vi "Close.vi"(8 "error in (no error)":errorcluster, 11 "IKA EUROSTAR Settings":T1) -> (0 "error out":errorcluster, 3 "IKA EUROSTAR Settings":T1)   [LabVIEW 2018, in "IKA EUROSTAR.lvlib"]
uses:
  IKA EUROSTAR.lvlib
  IKA EUROSTAR Settings.ctl
  support/Support Library.lvlib
panel:
  out "read buffer 2":string
  out "read buffer":string
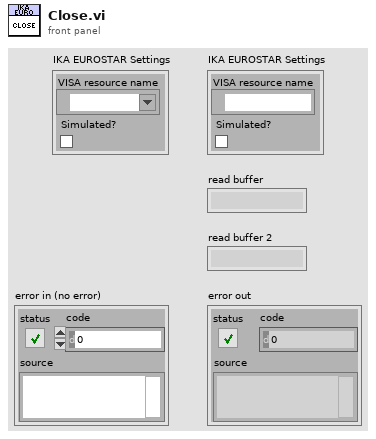
[diagram p1: front panel]
types:
  T1 = typedef "IKA EUROSTAR.lvlib/IKA EUROSTAR Settings.ctl" = cluster{"VISA resource name":refnum<visa-resource-name>, "Simulated?":bool}
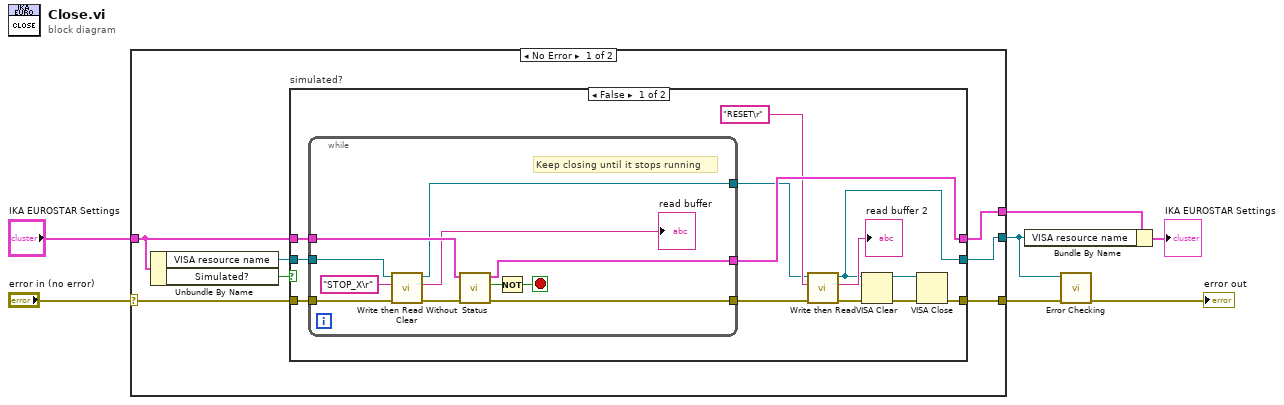
[diagram p0: block diagram]
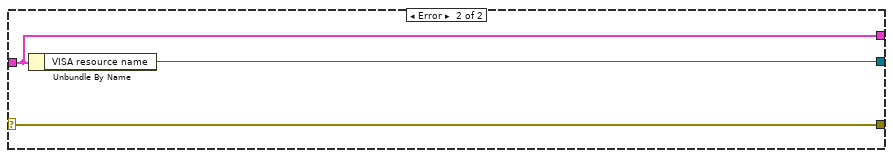
[diagram p3: hidden frame]
diagram:
  n1 = case shown="No Error" "error in (no error)" {
    selector: "error in (no error)" -> [w12 w44]
    tunnel: [w13 w44] -> w6
    tunnel: "IKA EUROSTAR Settings" -> [w9 w42]
    tunnel: [w10 w43] -> w4
    tunnel: [w8 w42] -> w3
    frame No Error {
      n2 = Unbundle By Name(w9) -> ("VISA resource name"=w11:refnum<visa-resource-name>, "Simulated?"=w14:bool)
      n3 = case "simulated?" shown="False" w14 {
        tunnel: [w27 w41] -> w13
        tunnel: w11 -> [w19 w40]
        tunnel: w12 -> [w21 w41]
        tunnel: [w18 w40] -> w10
        tunnel: w9 -> [w26 w39]
        tunnel: [w25 w39] -> w8
        frame False {
          n4 = while {
            tunnel: w26 -> [w35]
            tunnel: [w36] -> w25
            tunnel: [w28] -> w22
            tunnel: w21 -> [w31]
            tunnel: [w34] -> w20
            tunnel: w19 -> [w33]
            stop <- w38 stop-if-true
            # "Keep closing until it stops running"
            n5 = call "Write then Read Without Clear.vi"("error in"=w31, "write buffer"="STOP_X\r" ("string"), "VISA resource name in"=w33) -> ("error out"=w30:errorcluster, "read buffer"=→"read buffer":string, "VISA resource name out"=w28:refnum<visa-resource-name>)  [unwired: 5 in, 1 out]
            n6 = call "Status.vi"("error in (no error)"=w30, "IKA EUROSTAR Settings in"=w35) -> ("error out"=w34:errorcluster, "Running"=w37:bool, "IKA EUROSTAR Settings Out"=w36:T1)  [unwired: 4 in, 3 out]
            n7 = Not(x=w37) -> (.not. x?=w38:bool)
          }
          n8 = call "Write then Read.vi"("error in"=w20, "write buffer"="RESET\r" ("string"), "VISA resource name in"=w22) -> ("error out"=w17:errorcluster, "read buffer"=→"read buffer 2":string, "VISA resource name out"=w18:refnum<visa-resource-name>)  [unwired: 5 in, 1 out]
          n9 = VISA Clear(VISA resource name=w18, error in (no error)=w17) -> (VISA resource name out=w16:refnum<visa-resource-name>, error out=w15:errorcluster)
          n10 = VISA Close(VISA resource name=w16, error in (no error)=w15) -> (error out=w27:errorcluster)
        }
        frame True {
        }
      }
    }
    frame Error {
      n11 = Unbundle By Name(w42) -> ("VISA resource name"=w43:refnum<visa-resource-name>)
    }
  }
  n12 = Bundle By Name(cluster=w3, "VISA resource name"=w4) -> (→"IKA EUROSTAR Settings":T1)
  n13 = call "Error Checking.vi"("error in (no error)"=w6, "VISA resource name"=w4) -> ("error out"=→"error out":errorcluster)  [unwired: 7 in, 2 out]
